vi "SDCP SMF Transmitter and Receiver - Notifiers and Queues FGV.vi"() -> ()   [LabVIEW 2020]
uses:
  Typedefs/SDCP SMF logger - SMF with timestamp.ctl
panel:
  in  "Command":T1(ring)
  out "error out":errorcluster
  in  "error in (no error)":errorcluster
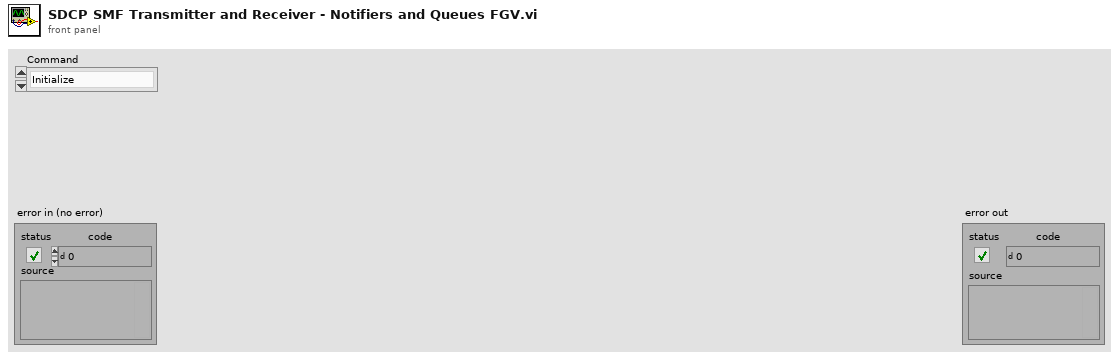
[diagram p1: front panel]
types:
  T1 = enum16{"Initialize", "Read notifiers", "Write notifiers", "Read queues", "Deinitialize"}
  T2 = typedef "SDCP SMF logger - SMF with timestamp.ctl" = cluster{"Bytes":u8[], "Checksum":bool, "Time (ms)":u32, "Tx/Rx":string}
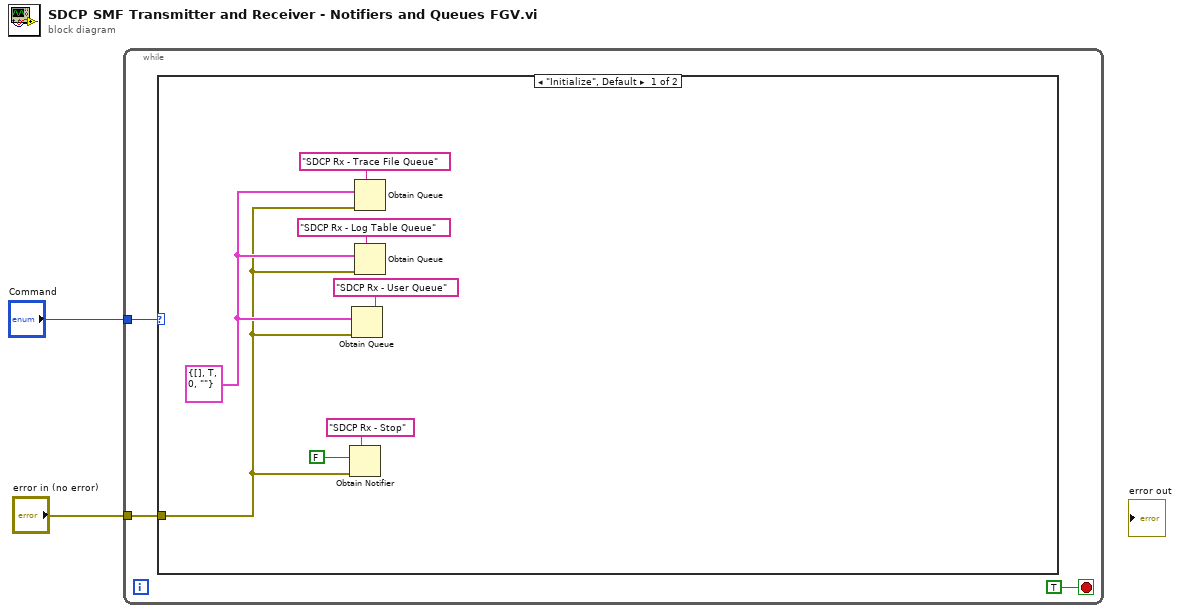
[diagram p0: block diagram]
diagram:
  n1 = while {
    tunnel: "error in (no error)" -> [w4]
    tunnel: "Command" -> [w3]
    stop <- TRUE stop-if-true
    n2 = case shown="\"Initialize\", Default" w3 {
      tunnel: w4 -> [w8 _]
      frame "Initialize", Default {
        w10 = T2 {"Bytes"=[], "Checksum"=TRUE, "Time (ms)"=0, "Tx/Rx"=""} ("SMF with timestamp")
        n3 = Obtain Notifier(name (unnamed)="SDCP Rx - Stop", notification data type=FALSE, error in (no error)=w8) -> ()  [unwired: 1 in, 3 out]
        n4 = Obtain Queue(name (unnamed)="SDCP Rx - User Queue", element data type=w10, error in (no error)=w8) -> ()  [unwired: 2 in, 3 out]
        n5 = Obtain Queue(name (unnamed)="SDCP Rx - Trace File Queue", element data type=w10, error in (no error)=w8) -> ()  [unwired: 2 in, 3 out]
        n6 = Obtain Queue(name (unnamed)="SDCP Rx - Log Table Queue", element data type=w10, error in (no error)=w8) -> ()  [unwired: 2 in, 3 out]
      }
      frame "Read notifiers" {
      }
    }
  }
